vi "Defer Front Panel.vi"() -> ()   [LabVIEW 2021]
panel:
  out "Numeric":i32
  out "Waveform Chart":dbl(graph)
  in  "stop":bool
  in  "Defer Panel Updates":bool
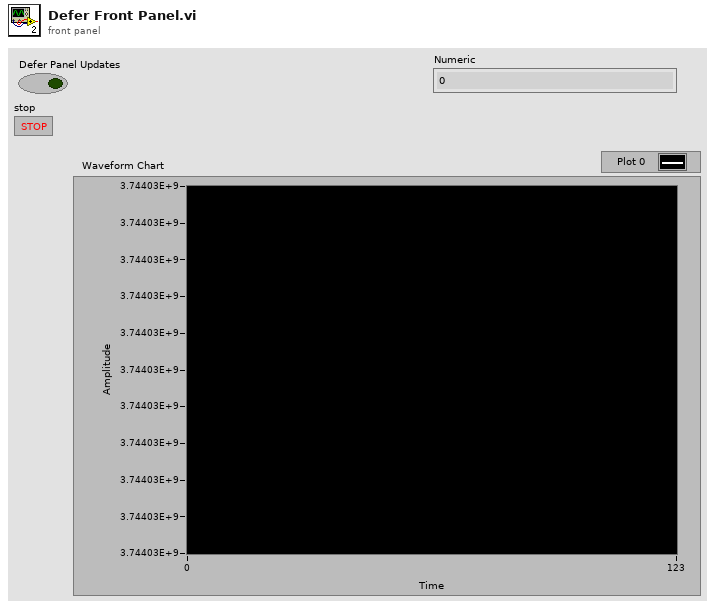
[diagram p1: front panel]
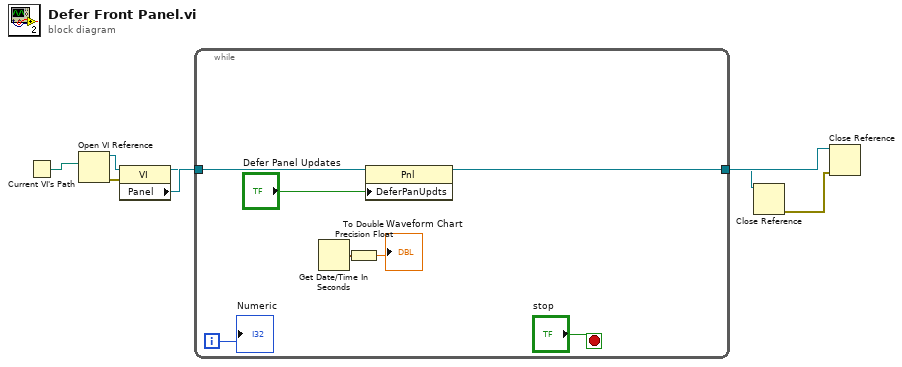
[diagram p0: block diagram]
diagram:
  n1 = Current VI's Path() -> (path=w1:path)
  n2 = Open VI Reference(vi path=w1) -> (vi reference=w7:refnum<vi>, error out=w5:errorcluster)  [unwired: 5 in]
  n3 = property class="VI"(reference=w7, error in=w5) -> (reference out=w4:refnum<vi>, "Panel"=w6:refnum<vi>)  [unwired: 1 out]
  n4 = while {
    tunnel: w6 -> [w14]
    tunnel: [w13] -> w3
    i -> [w11]
    stop <- "stop" stop-if-true
    n5 = Get Date/Time In Seconds() -> (seconds since 1Jan1904=w9:timestamp)
    n6 = To Double Precision Float(number=w9) -> (double precision float=→"Waveform Chart":dbl)
    n7 = property class="Pnl"(reference=w14, "DeferPanUpdts"="Defer Panel Updates") -> (reference out=w13:refnum<vi>)  [unwired: 1 in, 1 out]
    "Numeric" <- w11
  }
  n8 = Close Reference(reference=w3) -> (error out=w2:errorcluster)  [unwired: 1 in]
  n9 = Close Reference(reference=w4, error in (no error)=w2) -> ()  [unwired: 1 out]
